vi "Get Event Data.vi"(8 "error in (no error)":errorcluster, 11 "FSM.Edge in":refnum<class "FSM.Edge.lvclass">) -> (0 "error out":errorcluster, 2 "Event Data":T1, 3 "FSM.Edge out":refnum<class "FSM.Edge.lvclass">)   [LabVIEW 2015, in "FSM.Edge.lvclass"]
uses:
  FSM.Edge.lvclass
  FSM.Edge.lvclass/FSM.Edge.ctl
  FSM.Label/FSM.Label.lvclass/FSM.Label.ctl
  FSM.Label/Read Text.vi
  FSM.Label/FSM.Label.lvclass
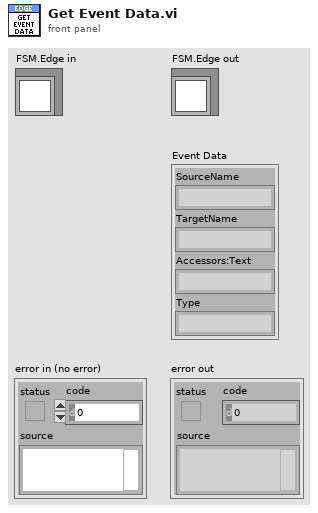
[diagram p1: front panel]
types:
  T1 = cluster{"SourceName":string, "TargetName":string, "Accessors:Text":string, "Type":string}
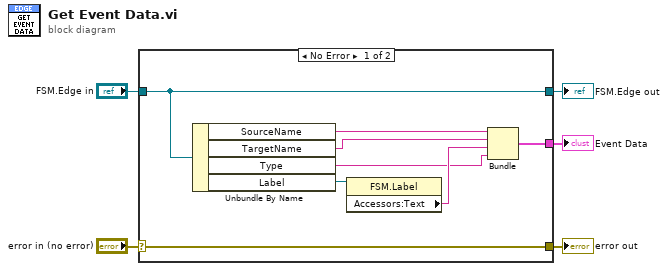
[diagram p0: block diagram]
diagram:
  n1 = case shown="No Error" "error in (no error)" {
    selector: "error in (no error)" -> [w13 w15]
    tunnel: [w13 w15] -> w4
    tunnel: [w12 w14] -> w2
    tunnel: "FSM.Edge in" -> [w12 w14]
    tunnel: [w6 _] -> w1
    frame No Error {
      n2 = Unbundle By Name(w12) -> ("SourceName"=w10:string, "TargetName"=w9:string, "Type"=w7:string, "Label"=w11:refnum<class "FSM.Label.lvclass">)
      n3 = property class="FSM.Label"(reference=w11) -> ("Accessors:Text"=w8:string)  [unwired: 1 in, 2 out]
      n4 = Bundle("SourceName"=w10, "TargetName"=w9, "Accessors:Text"=w8, "Type"=w7) -> (w6:T1)  [unwired: 1 in]
    }
    frame Error {
    }
  }
  "error out" <- w4
  "FSM.Edge out" <- w2
  "Event Data" <- w1
